vi "sv_Threshold Phases and Adjust T0.vi"(0 "Phases [1/cycle]":dbl[](array[numeric]), 1 "phase delay [1/cycle]":dbl, 2 "reset?":bool, 7 "dt":dbl, 9 "t0":timestamp) -> (4 "Phases [1/cycle]":dbl[](array[numeric]), 8 "dt out":dbl, 10 "t0 out":timestamp)   [LabVIEW 2017, in "SoundVib_ContSweptSine.lvlib"]
uses:
  <vilib>/addons/Sound and Vibration/svt_Continuous Swept Sine/SoundVib_ContSweptSine.lvlib
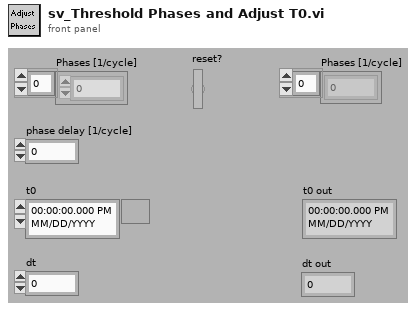
[diagram p1: front panel]
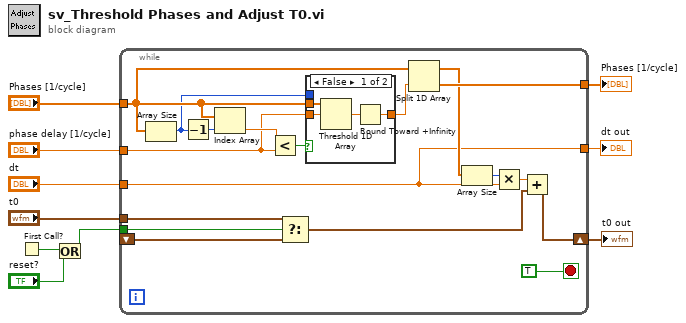
[diagram p0: block diagram]
diagram:
  n1 = First Call?() -> (First Call?: T/F=w6:bool)
  n2 = Or(x=w6, y="reset?") -> (x .or. y?=w4:bool)
  n3 = while {
    tunnel: "Phases [1/cycle]" -> [w15]
    tunnel: "phase delay [1/cycle]" -> [w11]
    tunnel: [w26] -> w3
    tunnel: "dt" -> [w18]
    tunnel: "t0" -> [w22]
    shift-right: [w17] -> w1
    shift-left: _ -> [w21]
    tunnel: w4 -> [w19]
    tunnel: [w18] -> w2
    stop <- TRUE stop-if-true
    n4 = Array Size(array=w15) -> (size(s)=w12:i32)
    n5 = Decrement(x=w12) -> (x-1=w16:i32)
    n6 = Index Array(array=w15, index=w16) -> (element=w14:dbl)
    n7 = Less?(x=w14, y=w11) -> (x < y?=w13:bool)
    n8 = Select(t=w22, s=w19, f=w21) -> (s? t:f=w20:timestamp)
    n9 = case shown="False" w13 {
      tunnel: [w31 w33] -> w27
      tunnel: w15 -> [w30 _]
      tunnel: w12 -> [_ w33]
      tunnel: w11 -> [w29 _]
      frame False {
        n10 = Threshold 1D Array(2:w29, 3:w30) -> (0:w32:dbl)  [unwired: 1 in]
        n11 = Round Toward +Infinity(x=w32) -> (ceil(x): smallest int >= x=w31:dbl)
      }
      frame True {
      }
    }
    n12 = Split 1D Array(array=w15, index=w27) -> (first subarray=w25:dbl[], second subarray=w26:dbl[])
    n13 = Array Size(array=w25) -> (size(s)=w24:i32)
    n14 = Multiply(x=w24, y=w18) -> (x*y=w23:dbl)
    n15 = Add(x=w23, y=w20) -> (x+y=w17:timestamp)
  }
  "Phases [1/cycle]" <- w3
  "dt out" <- w2
  "t0 out" <- w1
